vi "Set Routing Channel Error.vi"(6 "validation information in":T1, 8 "error in":errorcluster, 9 "routing channel error information":T2, 11 "routing channel in":T3 format="%.0x") -> (0 "error out":errorcluster, 1 "veristand error out":errorcluster, 3 "routing channel out":T3 format="%.0x", 4 "validation information out":T1)   [LabVIEW 2020, in "Routing and Faulting Scripting.lvlib"]
uses:
  Routing and Faulting Scripting.lvlib
  <vilib>/NI VeriStand/Custom Device API/Custom Device Item Ref.ctl
  Routing Channel Error Information.ctl
  Validation/Validation Information.ctl
  <vilib>/NI VeriStand/Custom Device API/Custom Device API.lvlib
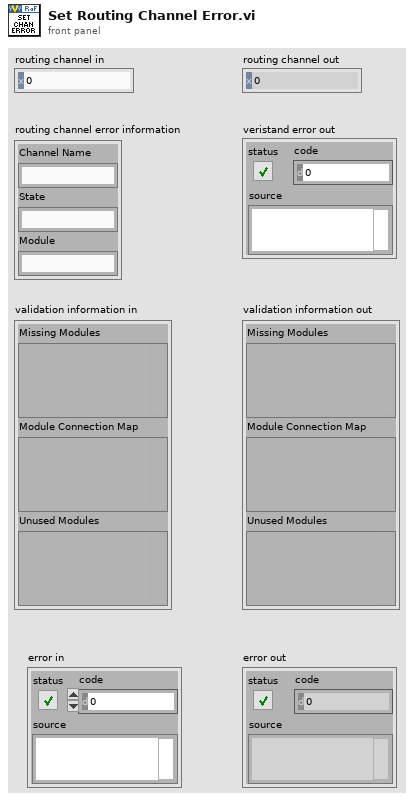
[diagram p1: front panel]
types:
  T1 = typedef "Routing and Faulting Scripting.lvlib/Validation Information.ctl" = cluster{"Missing Modules":variant, "Module Connection Map":variant, "Unused Modules":variant}
  T2 = typedef "Routing and Faulting Scripting.lvlib/Routing Channel Error Information.ctl" = cluster{"Channel Name":string, "State":string, "Module":string}
  T3 = typedef "Custom Device API.lvlib/Custom Device Item Ref.ctl" = u64
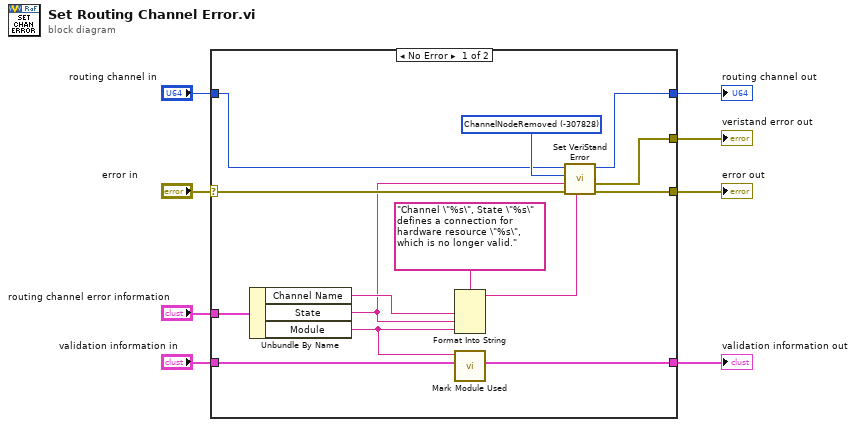
[diagram p0: block diagram]
diagram:
  n1 = case shown="No Error" "error in" {
    selector: "error in" -> [w13 w25]
    tunnel: "routing channel in" -> [w19 w24]
    tunnel: [w18 w24] -> w7
    tunnel: "routing channel error information" -> [w17 _]
    tunnel: [w15 w25] -> w5
    tunnel: [w14 _] -> w4
    tunnel: "validation information in" -> [w12 w23]
    tunnel: [w11 w23] -> w1
    frame No Error {
      w21 = -307828 items=["Success"=0, "NoProjectOpen"=-307992, "SequenceCompileError"=-307988, "SessionAlreadyDeployed"=-307984, "SessionNotDeployed"=-307982, "SequenceNotFoundInSession"=-307981, "StimulusProfileSessionLocked"=-307980, "EmptyNodeName"=-307930, "NodeAlreadyExistsByName"=-307926, "NumberOfCoefficientsOutOfRange"=-307884, "DownloadFileError"=-307872, "IncorrectLogFileName"=-307871, "LogTriggerConditionSyntaxError"=-307868, "DuplicateLogSessionName"=-307867, "LogSessionNotFound"=-307865, "ChannelLengthMismatch"=-307830, "NodeNotFoundDuringCompile"=-307829, "ChannelNodeRemoved"=-307828, "NotAChannel"=-307825, "NotAWaveform"=-307824, "STIFileError"=-307784, "DependenciesCycle"=-307783, "ChannelNotFoundInLogFile"=-307782, "ChannelGroupNotFoundInLogFile"=-307781, "GatewayNotOnLocalhost"=-307780, "NotEnoughDynamicDataSharingSpace"=-307738, "TargetMissingDataSharingDevice"=-307737, "ChannelMappingsSizeMismatch"=-307728, "DuplicateChannelAliasMappings"=-307711, "NotAnInlineCustomDevice"=-307710, "IncompatibleModel"=-307703, "ModelDimensionMismatch"=-307702, "SLSCChassisLoadFailed"=-307691, "TargetDisabled"=-307689, "MismatchedLengths"=-307687, "TargetInvalid"=-307686, "ParameterNotFound"=-307685, "ServerPortAlreadyInUse"=-307684, "TargetDisconnected"=-307682, "ServiceConfigurationFile"=-307681, "ModelParameterFileParseError"=-307680, "NoActionRequired"=-307677, "InputParameterInvalid"=-307676, "HostRunningDifferentSystemDefinition"=-307671, "ChannelNotScalable"=-307668, "ChannelCannotBeFaulted"=-307666, "ChannelNotWritable"=-307665, "ChannelNotReadable"=-307664, "Timeout"=-307663, "NodeNotFound"=-307662, "SystemDefinitionDeploymentFailure"=-307661, "SystemDefinitionDeploymentTimeout"=-307660, "EmptyPassword"=-307659, "SystemDefinitionAlreadyActive"=-307658, "InvalidConfigurationPassword"=-307657, "NoSystemDefinitionLoaded"=-307656, "ComponentNotAvailable"=-307655, "NotDeployed"=-307654, "InvalidFile"=-307653, "FailedServerConnection"=-307652, "FunctionNotSupported"=-307651, "UnexpectedError"=-307650, "UnmappedAlias"=-307617, "InvalidStreamConditionForDataType"=-307554, "WaveformDataTypeMismatch"=-307553, "InvalidDaqPluginFile"=-307526, "FileVersionUnsupported"=-307525] ("NationalInstruments.VeriStand.ErrorCode")
      n2 = Unbundle By Name(w17) -> ("Channel Name"=w16:string, "State"=w9:string, "Module"=w10:string)
      n3 = Format Into String(format string="Channel \"%s\", State \"%s\" defines a connection for hardware resource \"%s\", which is no longer valid.", w16, w9, w10) -> (resulting string=w20:string)  [unwired: 2 in, 1 out]
      n4 = call "Mark Module Used.vi"("validation information in"=w12, "module path"=w10) -> ("validation information out"=w11:T1)  [unwired: 8 in, 1 out]
      n5 = call "Set VeriStand Error.vi"("message"=w20, "error in"=w13, "key"=w9, "error code"=w21, "item in"=w19) -> ("error out"=w15:errorcluster, "veristand error out"=w14:errorcluster, "item out"=w18:T3)  [unwired: 4 in]
    }
    frame Error {
    }
  }
  "routing channel out" <- w7
  "error out" <- w5
  "veristand error out" <- w4
  "validation information out" <- w1
